vi "Init.vi"(8 "error in":errorcluster, 11 "IInitialize in":refnum<class "IInitialize.lvclass">) -> (0 "error out":errorcluster, 3 "IInitialize out":refnum<class "IInitialize.lvclass">)   [LabVIEW 2025, in "IInitialize.lvclass"]
uses:
  IInitialize.lvclass
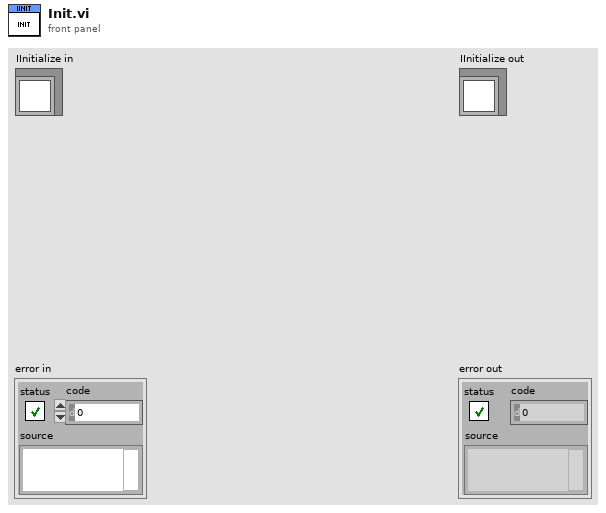
[diagram p1: front panel]
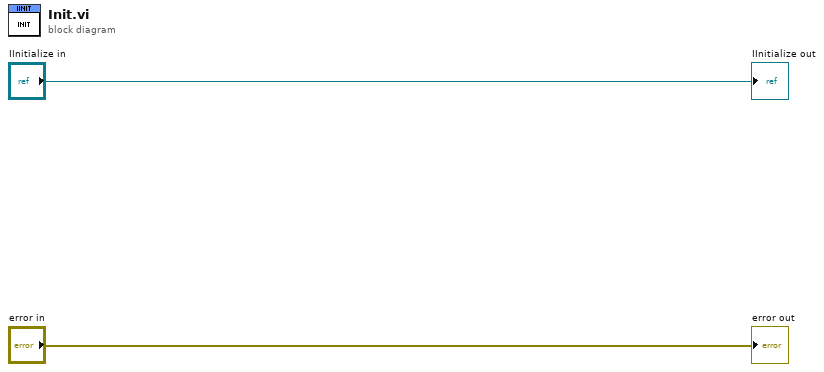
[diagram p0: block diagram]
diagram:
  "error out" <- "error in"
  "IInitialize out" <- "IInitialize in"
